vi "Read TDMS-Data.vi"(8 "error in (no error)":errorcluster, 11 "Update TDMS-Data Msg in":refnum<class "Update TDMS-Data Msg.lvclass">) -> (0 "error out":errorcluster, 2 "BNT_TDMS.lvlib:TDMS-Data.lvclass":refnum<class "TDMS-Data.lvclass">, 3 "Update TDMS-Data Msg out":refnum<class "Update TDMS-Data Msg.lvclass">)   [LabVIEW 2017, in "BNT_TDMS.lvlib" / "Update TDMS-Data Msg.lvclass"]
uses:
  Update TDMS-Data Msg.lvclass
  TDMSData/TDMS-Data.lvclass
  Update TDMS-Data Msg.lvclass/Update TDMS-Data Msg.ctl
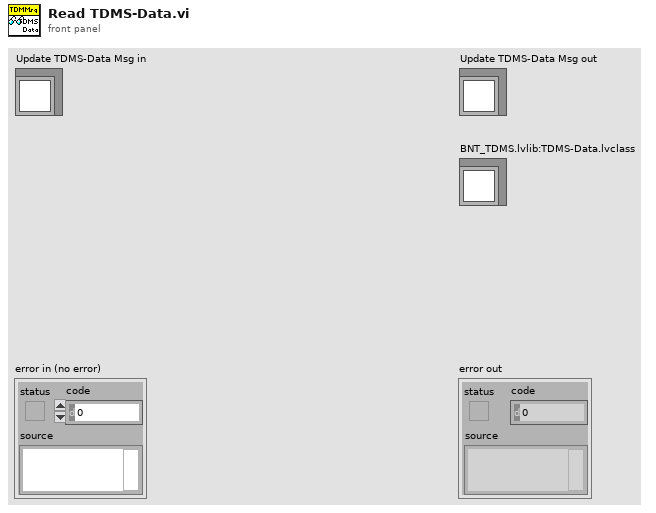
[diagram p1: front panel]
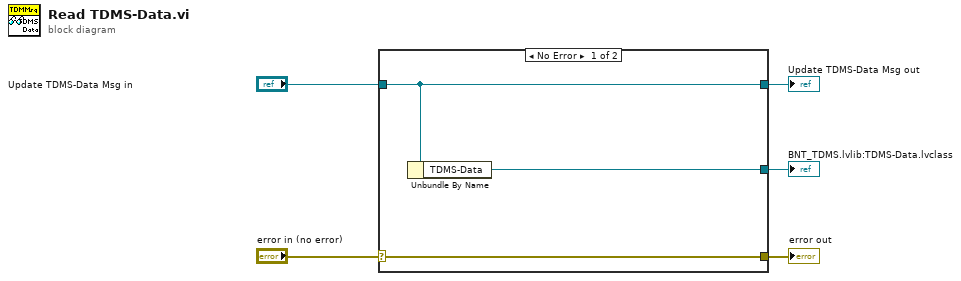
[diagram p0: block diagram]
diagram:
  n1 = case shown="No Error" "error in (no error)" {
    selector: "error in (no error)" -> [w8 w9]
    tunnel: [w8 w9] -> w4
    tunnel: [w7 w10] -> w2
    tunnel: "Update TDMS-Data Msg in" -> [w7 w10]
    tunnel: [w6 _] -> w1
    frame No Error {
      n2 = Unbundle By Name(w7) -> ("TDMS-Data"=w6:refnum<class "TDMS-Data.lvclass">)
    }
    frame Error {
    }
  }
  "error out" <- w4
  "Update TDMS-Data Msg out" <- w2
  "BNT_TDMS.lvlib:TDMS-Data.lvclass" <- w1
